vi "Get ProjectItem Descendants (with Type).vi"(7 "Type":string, 8 "error in (no error)":errorcluster, 11 "ProjectItem in":refnum<vi>) -> (0 "error out":errorcluster, 2 "All Descendents":refnum<vi>[](array[refnum]), 3 "ProjectItem out":refnum<vi>)   [LabVIEW 2020, in "gRPC Scripting Tools.lvlib"]
uses:
  gRPC Scripting Tools.lvlib
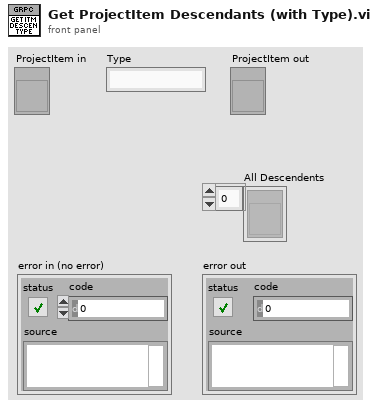
[diagram p1: front panel]
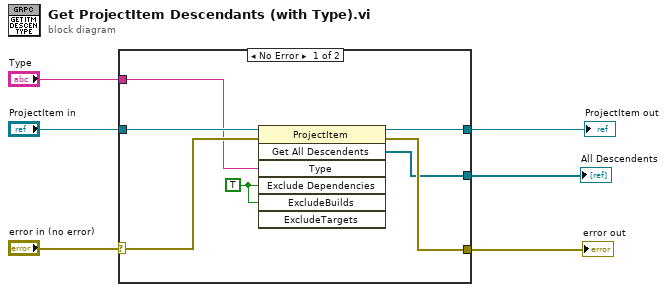
[diagram p0: block diagram]
diagram:
  n1 = case shown="No Error" "error in (no error)" {
    selector: "error in (no error)" -> [w9 w14]
    tunnel: "ProjectItem in" -> [w13 w15]
    tunnel: [w11 w14] -> w5
    tunnel: [w10 _] -> w4
    tunnel: [w8 w15] -> w2
    tunnel: "Type" -> [w7 _]
    frame No Error {
      w12 = TRUE ("ExcludeDependencies")
      n2 = invoke class="ProjectItem" method="Get All Descendents"(reference=w13, error in=w9, "Type"=w7, "Exclude Dependencies"=w12, "ExcludeBuilds"=w12) -> (reference out=w8:refnum<vi>, error out=w11:errorcluster, "All Descendents"=w10:refnum<vi>[])  [unwired: 2 in, 4 out]
    }
    frame Error {
    }
  }
  "error out" <- w5
  "All Descendents" <- w4
  "ProjectItem out" <- w2
